vi "ABR-Read Header.vi"(0 "Path":path, 11 "error in":errorcluster) -> (4 "Path (thru)":path, 8 "Header":T1={"RUN-"=0, "SW FREQ:"=0.0, "# AVERAGES:"=0, "REP RATE (/sec):"=0.0, "SAMPLE (µsec):"=0.0, "CHAMBER-"="", "CFTS Version: "="", "LEVELS:"=[], "Date"=timestamp(0 s since 1904-01-01), "Threshold:"=nan}, 15 "error out":errorcluster)   [LabVIEW 2020]
uses:
  TypeDefs/ABR-Data Header.ctl
  <vilib>/regexp/Match Regular Expression.xnode
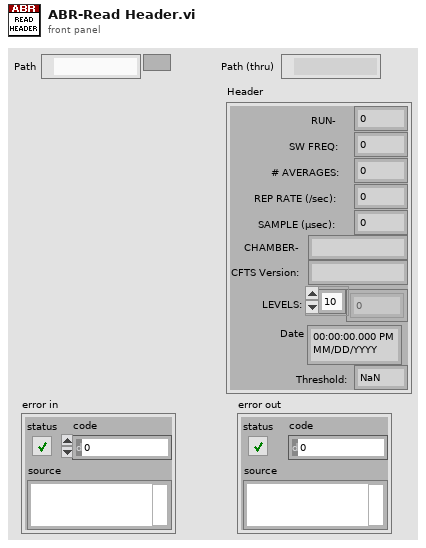
[diagram p1: front panel]
types:
  T1 = typedef "ABR-Data Header.ctl" = cluster{"RUN-":i32, "SW FREQ:":dbl, "# AVERAGES:":i32, "REP RATE (/sec):":dbl, "SAMPLE (µsec):":dbl, "CHAMBER-":string, "CFTS Version: ":string, "LEVELS:":dbl[], "Date":timestamp, "Threshold:":dbl}
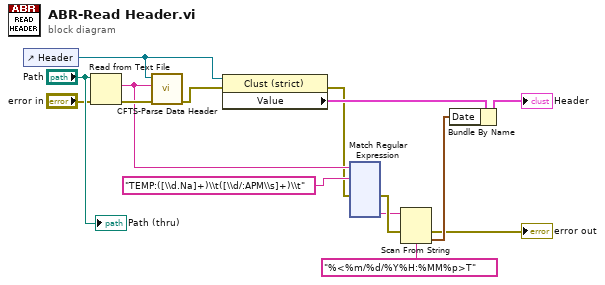
[diagram p0: block diagram]
diagram:
  n1 = control-ref of="Header"() -> (w6:refnum<vi>)
  n2 = Read from Text File(file (use dialog)="Path", error in="error in") -> (text=w11:string, error out=w14:errorcluster)  [unwired: 2 in, 2 out]
  n3 = call "CFTS-Parse Data Header.vi"("error in (no error)"=w14, "Header string"=w11, "Cluster Ref In"=w6) -> ("error out"=w13:errorcluster)  [unwired: 7 in, 1 out]
  n4 = property class="Clust (strict)"(reference=w6, error in=w13) -> (error out=w5:errorcluster, "Value"=w9:T1)  [unwired: 1 out]
  n5 = xnode "Match Regular Expression"("input string"=w11, "regular expression"="TEMP:([\\d.Na]+)\\t([\\d/:APM\\s]+)\\t" ("string"), "error in"=w5) -> ("error out"=w4:errorcluster, "submatch 2"=w2:string)  [unwired: 3 in, 5 out]
  n6 = Scan From String(format string="%<%m/%d/%Y%H:%MM%p>T", input string=w2, error in=w4) -> (error out=→"error out":errorcluster, output 1=w7:timestamp)  [unwired: 2 in, 2 out]
  n7 = Bundle By Name(cluster=w9, "Date"=w7) -> (→"Header":T1)
  "Path (thru)" <- "Path"
